vi "CLSUIP_ParentChangedEventGlobal.vi"() -> ()   [LabVIEW 2021]
uses:
  <resource>/Framework/Providers/LVClassLibrary/CLSUIP_ParentChangedData.ctl
panel:
  out "Parent Changed Event":refnum<user-event>
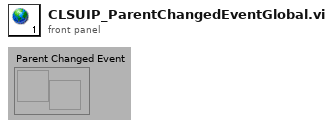
[diagram p1: front panel]
diagram:
